vi "Master Setup Startup Procedure.vi"(8 "Queue (in)":refnum<queue>, 10 "Don't Wait for Channel Update":bool) -> (0 "File Operations":T1, 1 "Run Time System":bool, 3 "Master Event Registration Refnum":refnum<event-registration>)   [LabVIEW 2017]
uses:
  Setup File Operations/File Operation with History.ctl
panel:
  out "Loop 3":i32
  out "Not a Valid Reference (Update Channel Rings)":bool
  out "Not a Valid Reference (Update Channels)":bool
  out "Not a Valid Reference (Master Save)":bool
  out "Not a Valid Reference (Master Open)":bool
  out "Not a Valid Reference (Master Exit)":bool
  out "Loop 2":i32
  out "Loop 1":i32
  out "error out":errorcluster
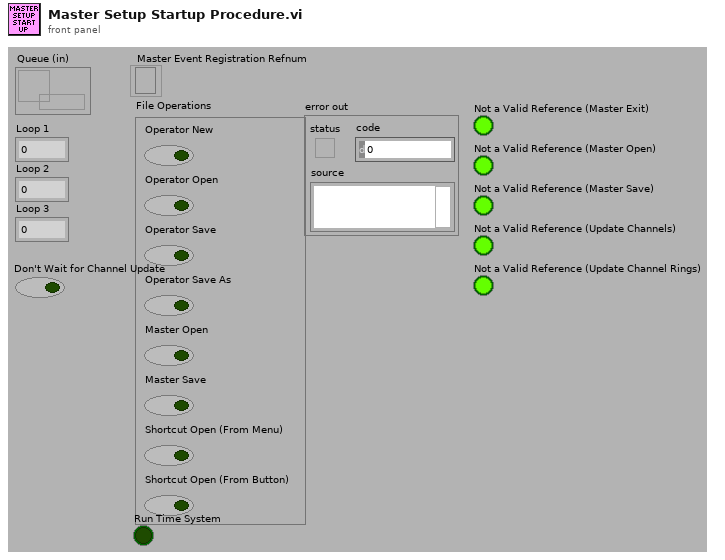
[diagram p1: front panel]
types:
  T1 = typedef "File Operation with History.ctl" = cluster{"Operator New":bool, "Operator Open":bool, "Operator Save":bool, "Operator Save As":bool, "Master Open":bool, "Master Save":bool, "Shortcut Open (From Menu)":bool, "Shortcut Open (From Button)":bool}
  T2 = enum32{"invalid app kind", "Development System", "Run Time System", "Student Edition", "Embedded LabVIEW", "Evaluation", "Custom"}
  T3 = cluster{"Master Exit":bool, "Master Open":bool, "Master Save":bool, "Update Channels":bool, "Update Channel Rings":bool}
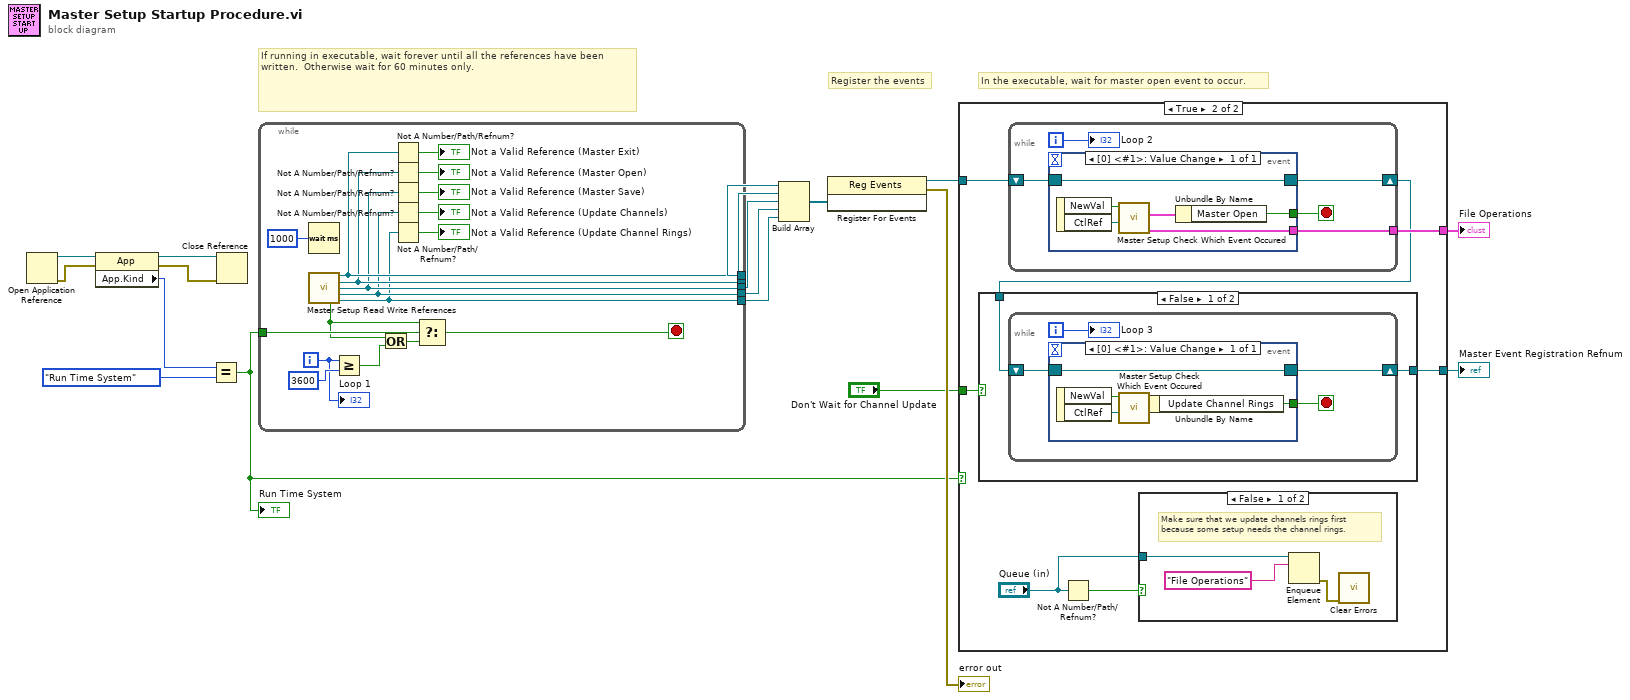
[diagram p0: block diagram]
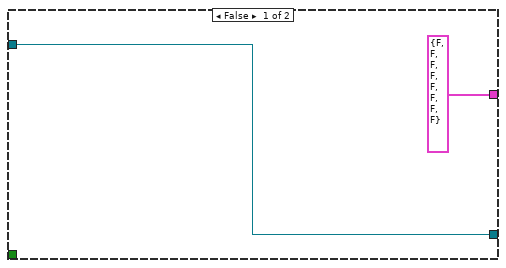
[diagram p2: hidden frame]
diagram:
  # "In the executable, wait for master open event to occur."
  # "Register the events"
  # "If running in executable, wait forever until all the references have been written.  Otherwise wait for 60 minutes only."
  n1 = Open Application Reference() -> (0:w17:errorcluster, 3:w18:refnum<vi>)  [unwired: 4 in]
  n2 = property class="App"(reference=w18, error in=w17) -> (reference out=w16:refnum<vi>, error out=w13:errorcluster, "App.Kind"=w15:T2)
  n3 = Equal?(x=w15, y=T2."Run Time System") -> (x = y?=w2:bool)
  "Run Time System" <- w2
  n4 = Close Reference(reference=w16, error in (no error)=w13) -> ()  [unwired: 1 out]
  n5 = while {
    tunnel: w2 -> [w34]
    tunnel: [w27] -> w6
    tunnel: [w26] -> w11
    tunnel: [w25] -> w10
    tunnel: [w24] -> w7
    tunnel: [w28] -> w8
    i -> [w29]
    stop <- w33 stop-if-true
    n6 = Wait (ms)(milliseconds to wait=u32 1000) -> ()  [unwired: 1 out]
    n7 = call "Master Setup Read Write References.vi"() -> ("Master Exited (out)"=w28:refnum<vi>, "Master Open (out)"=w27:refnum<vi>, "Master Save (out)"=w26:refnum<vi>, "Update Channels (out)"=w25:refnum<vi>, "Valid References"=w32:bool, "Update Channel Rings (out)"=w24:refnum<vi>)  [unwired: 10 in]
    n8 = Greater Or Equal?(x=w29, y=3600) -> (x >= y?=w31:bool)
    n9 = Or(x=w32, y=w31) -> (x .or. y?=w30:bool)
    n10 = Not A Number/Path/Refnum?(number/path/refnum=w28) -> (NaN/Path/Refnum?=→"Not a Valid Reference (Master Exit)":bool)
    n11 = Not A Number/Path/Refnum?(number/path/refnum=w27) -> (NaN/Path/Refnum?=→"Not a Valid Reference (Master Open)":bool)
    n12 = Not A Number/Path/Refnum?(number/path/refnum=w26) -> (NaN/Path/Refnum?=→"Not a Valid Reference (Master Save)":bool)
    n13 = Not A Number/Path/Refnum?(number/path/refnum=w25) -> (NaN/Path/Refnum?=→"Not a Valid Reference (Update Channels)":bool)
    n14 = Not A Number/Path/Refnum?(number/path/refnum=w24) -> (NaN/Path/Refnum?=→"Not a Valid Reference (Update Channel Rings)":bool)
    n15 = Select(t=w32, s=w34, f=w30) -> (s? t:f=w33:bool)
    "Loop 1" <- w29
  }
  n16 = Build Array(w8, w6, w11, w10, w7) -> (w12:refnum<vi>[])
  n17 = register-events(w12) -> (reference out=w5:refnum<event-registration>, error out=→"error out":errorcluster)  [unwired: 2 in]
  n18 = case shown="True" w2 {
    tunnel: w5 -> [w38 w42]
    tunnel: [w38 w39] -> w3
    tunnel: [T1 {"Operator New"=FALSE, "Operator Open"=FALSE, "Operator Save"=FALSE, "Operator Save As"=FALSE, "Master Open"=FALSE, "Master Save"=FALSE, "Shortcut Open (From Menu)"=FALSE, "Shortcut Open (From Button)"=FALSE} ("File Operations") w43] -> w4
    tunnel: "Don't Wait for Channel Update" -> [_ w41]
    frame False {
    }
    frame True {
      n19 = while {
        shift-right: [w61] -> w40
        shift-left: w42 -> [w62]
        tunnel: [w60] -> w43
        i -> [w58]
        stop <- w59 stop-if-true
        n20 = event shown="[0] <#1>: Value Change" {
          selector: w62 -> [w67]
          dyn-events: [w67] -> w61
          timeout: _ -> [_]
          tunnel: [w66] -> w60
          tunnel: [w64] -> w59
          event Value Change {
            n21 = event-data() -> ("NewVal"=w68:bool, "CtlRef"=w63:refnum<vi>)  [unwired: 1 in]
            n22 = call "Master Setup Check Which Event Occured.vi"("CtlRef"=w63, "NewVal"=w68) -> ("File Operations"=w66:T1, "Event Occurred"=w65:T3)  [unwired: 3 in, 1 out]
            n23 = Unbundle By Name(w65) -> ("Master Open"=w64:bool)
          }
        }
        "Loop 2" <- w58
      }
      n24 = case shown="False" w41 {
        tunnel: w40 -> [w47 w57]
        tunnel: [w46 w57] -> w39
        frame False {
          n25 = while {
            shift-right: [w50] -> w46
            shift-left: w47 -> [w51]
            i -> [w48]
            stop <- w49 stop-if-true
            n26 = event shown="[0] <#1>: Value Change" {
              selector: w51 -> [w55]
              dyn-events: [w55] -> w50
              timeout: _ -> [_]
              tunnel: [w53] -> w49
              event Value Change {
                n27 = event-data() -> ("NewVal"=w56:bool, "CtlRef"=w52:refnum<vi>)  [unwired: 1 in]
                n28 = call "Master Setup Check Which Event Occured.vi"("CtlRef"=w52, "NewVal"=w56) -> ("Event Occurred"=w54:T3)  [unwired: 3 in, 2 out]
                n29 = Unbundle By Name(w54) -> ("Update Channel Rings"=w53:bool)
              }
            }
            "Loop 3" <- w48
          }
        }
        frame True {
        }
      }
      n30 = Not A Number/Path/Refnum?(number/path/refnum="Queue (in)") -> (NaN/Path/Refnum?=w44:bool)
      n31 = case shown="False" w44 {
        tunnel: "Queue (in)" -> [w69 _]
        frame False {
          # "Make sure that we update channels rings first because some setup needs the channel rings."
          n32 = Enqueue Element(queue=w69, element="File Operations") -> (error out=w70:errorcluster)  [unwired: 2 in, 2 out]
          n33 = call <vilib>:"Clear Errors.vi"("error in (no error)"=w70) -> ()  [unwired: 5 in, 2 out]
        }
        frame True {
        }
      }
    }
  }
  "File Operations" <- w4
  "Master Event Registration Refnum" <- w3
